vi "Snapshot.vi"(6 "Dest Format":string(combo)="{6fddc324-4e03-4bfe-b185-3d77768dc90e}", 9 "Stop Ref":refnum<vi>, 10 "Value":T3, 11 "Refnum in":T2) -> (3 "headers":string)   [LabVIEW 2016]
uses:
  cgi_string.ctl
  <vilib>/httpClient/ClientHandle.ctl
  <vilib>/vision/Image Controls.llb/IMAQ Image.ctl
  <vilib>/httpClient/LabVIEWHTTPClient.lvlib
panel:
  in  "stop":bool
  out "Dest Format":string(combo)="{6fddc324-4e03-4bfe-b185-3d77768dc90e}"
  out "Image":T1(plugin-control)
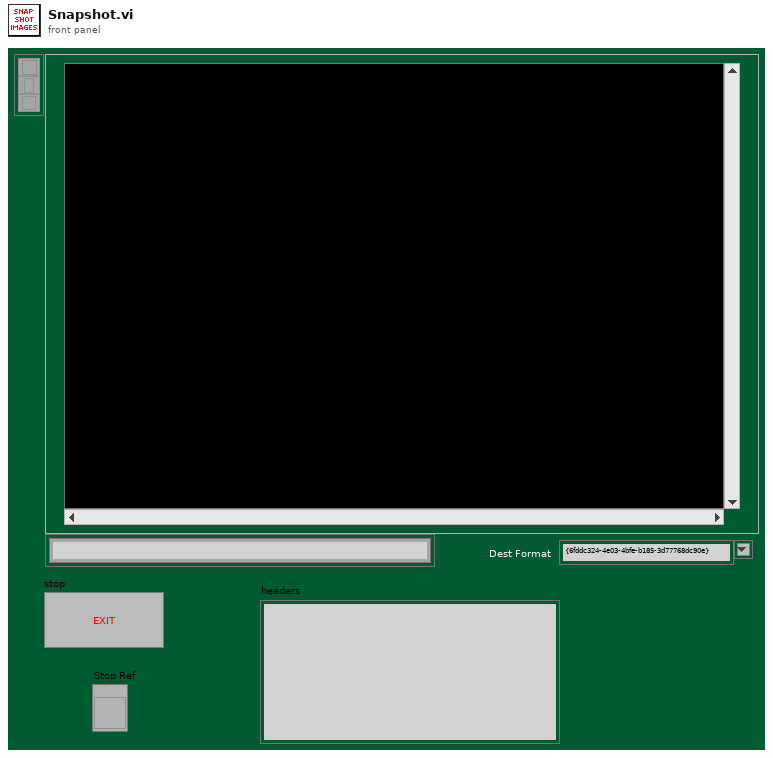
[diagram p1: front panel]
types:
  T1 = typedef "IMAQ Image.ctl" = refnum<image>
  T2 = typedef "LabVIEWHTTPClient.lvlib/ClientHandle.ctl" = refnum<k1>
  T3 = typedef "cgi_string.ctl" = string
  T4 = typedef "Image Type" = u32
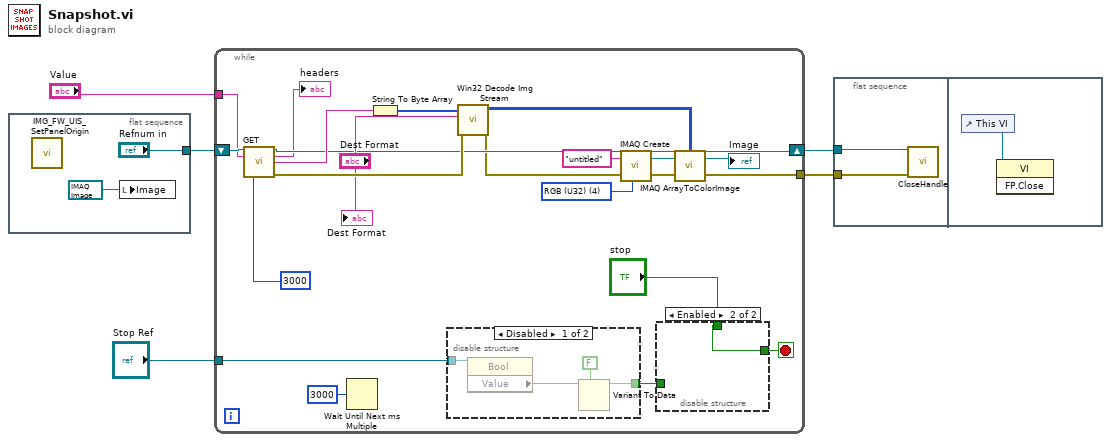
[diagram p0: block diagram]
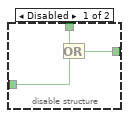
[diagram p3: hidden frame]
diagram:
  n1 = flat-sequence {
    tunnel: ["Refnum in"] -> w5
    frame #0 {
      n2 = call "IMG_FW_UIS_SetPanelOrigin.vi"() -> ()  [unwired: 11 in, 1 out]
      n3 = local write "Image"(T1 refnum ("New Image")) -> ()
    }
  }
  n4 = while {
    tunnel: [w24] -> w4
    tunnel: "Value" -> [w21]
    shift-right: [w23] -> w3
    shift-left: w5 -> [w29]
    tunnel: "Stop Ref" -> [w12]
    stop <- w13 stop-if-true
    w19 = T4 4 items=["Grayscale (U8)", "Grayscale (I16)", "Grayscale (SGL)", "Complex (CSG)", "RGB (U32)", "HSL (U32)", "RGB (U64)", "Grayscale (U16)"] ("Image Type")
    n5 = call <vilib>:"GET.vi"("client handle"=w29, "url"=w21, "timeout (10000)"=u32 3000 ("millisecond multiple")) -> ("client handle out"=w23:T2, "headers"=→"headers":string, "body"=w26:string, "error out"=w27:errorcluster)  [unwired: 9 in]
    n6 = Wait Until Next ms Multiple(millisecond multiple=u32 3000) -> ()  [unwired: 1 out]
    n7 = String To Byte Array(string=w26) -> (unsigned byte array=w28:u8[])
    n8 = disable-structure shown="Disabled" {
      disable-tunnel: w12 -> [w33 _]
      disable-tunnel: [w30 _] -> w11
      frame Disabled {
        n9 = property class="Bool"(reference=w33) -> ("Value"=w32:variant)  [unwired: 1 in, 2 out]
        n10 = Variant To Data(type=FALSE, Variant=w32) -> (data=w30:bool)  [unwired: 1 in, 1 out]
      }
      frame Enabled {
      }
    }
    n11 = call "Win32 Decode Img Stream.vi"("error in (no error)"=w27, "Dest Format"="Dest Format", "Image Data"=w28) -> ("error out"=w16:errorcluster, "Dest"=w14:u32[][])  [unwired: 4 in, 3 out]
    n12 = call "IMAQ Create"("Image Name"="untitled", "Image Type"=w19, "error in (no error)"=w16) -> ("New Image"=w20:T1, "error out"=w17:errorcluster)  [unwired: 2 in]
    n13 = disable-structure shown="Enabled" {
      disable-tunnel: [w36 w37] -> w13
      disable-tunnel: w11 -> [w35 _]
      disable-tunnel: "stop" -> [w34 w37]
      frame Disabled {
        n14 = Or(x=w34, y=w35) -> (x .or. y?=w36:bool)
      }
      frame Enabled {
      }
    }
    n15 = call "IMAQ ArrayToColorImage"("Image Pixels (U32)"=w14, "Image"=w20, "error in (no error)"=w17) -> ("Image Out"=→"Image":T1, "error out"=w24:errorcluster)  [unwired: 2 in]
    "Dest Format" <- "Dest Format"
  }
  n16 = flat-sequence {
    tunnel: w4 -> [w39]
    tunnel: w3 -> [w38]
    frame #0 {
      n17 = call <vilib>:"CloseHandle.vi"("client handle"=w38, "error in (no error)"=w39) -> ()  [unwired: 13 in, 1 out]
    }
    frame #1 {
      n18 = control-ref of="This VI"() -> (w40:refnum<vi>)
      n19 = invoke class="VI" method="FP.Close"(reference=w40) -> ()  [unwired: 2 in, 3 out]
    }
  }
